vi "continuous move V1.2.vi"() -> ()   [LabVIEW 2019]
uses:
  position cluster.ctl
  move array and radius.ctl
panel:
  in  "Position in":T1
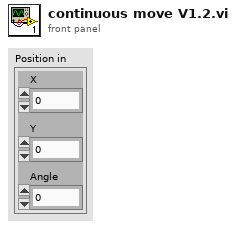
[diagram p1: front panel]
types:
  T1 = typedef "position cluster.ctl" = cluster{"X":dbl, "Y":dbl, "Angle":dbl}
  T2 = typedef "move array and radius.ctl" = cluster{"X":dbl, "Y":dbl, "R":dbl}[]
  T3 = typedef "move array.ctl" = cluster{"X":dbl, "Y":dbl}[]
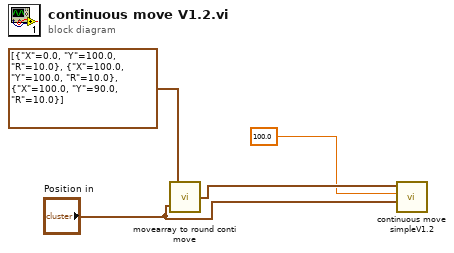
[diagram p0: block diagram]
diagram:
  n1 = call "movearray to round conti move.vi"("Position in"="Position in", "move array"=T2 [{"X"=0.0, "Y"=100.0, "R"=10.0}, {"X"=100.0, "Y"=100.0, "R"=10.0}, {"X"=100.0, "Y"=90.0, "R"=10.0}]) -> ("move array out"=w4:T3)
  n2 = call "continuous move simpleV1.2.vi"("Position"="Position in", "Speed"=100.0, "Array"=w4) -> ()  [unwired: 7 in, 2 out]
